vi "CSM - Argument Type.vi"(5 "Arguments":string) -> (1 "Argument Type":string, 2 "Arguments (Dup)":string)   [LabVIEW 2017, in "CSM Shared.lvlib"]
doc: "Extracts the parameter encoding type tag from the encoded argument string.\n\n> [!NOTE] \n> <b>CSM Argument Type</b>\n>\n> In CSM, all arguments and return values are presented in string format, but they can carry any data type underneath. Therefore, the sender must encode first, and the receiver must decode afterwards. For example, CSM has a built-in HEXSTR encoding scheme, and custom codecs can also be extended as needed. To facilitate the identification of the encoding method, it is recommended to write the encoded argument in the format `<Argument Type> STRING FORMAT ARGUMENT`. Use the CSM - Argument Type VI to extract the type tag and select the corresponding decoding function accordingly.\n\n\n-- <b>Controls</b> --\n- <b>Arguments</b>: Argument string.\n\n-- <b>Indicators</b> --\n- <b>Argument Type</b>: Encoding type tag of the argument string.\n- <b>Arguments (Dup)</b>: A copy of the input argument string."
uses:
  CSM Shared.lvlib
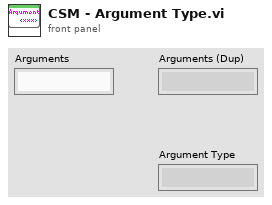
[diagram p1: front panel]
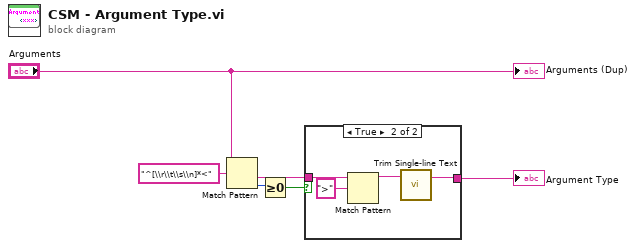
[diagram p0: block diagram]
diagram:
  n1 = Match Pattern(string="Arguments", regular expression="^[\\r\\t\\s\\n]*<") -> (after substring=w3:string, offset past match=w4:i32)  [unwired: 1 in, 2 out]
  n2 = Greater Or Equal To 0?(x=w4) -> (x >= 0?=w5:bool)
  n3 = case shown="True" w5 {
    tunnel: w3 -> [_ w9]
    tunnel: [_ w7] -> w6
    frame False {
    }
    frame True {
      n4 = Match Pattern(string=w9, regular expression=">") -> (before substring=w8:string)  [unwired: 1 in, 3 out]
      n5 = call "Trim Single-line Text.vi"("single-line text"=w8) -> ("trimed text"=w7:string)  [unwired: 2 in]
    }
  }
  "Argument Type" <- w6
  "Arguments (Dup)" <- "Arguments"
